vi "Get Label Prepend Append.vi"(8 "error in (no error)":errorcluster, 11 "CConfig Variant Accessor in":refnum<class "CConfig Variant Accessor.lvclass">) -> (0 "error out":errorcluster, 1 "Label Append":string, 2 "Label Prepend":string, 3 "CConfig Variant Accessor out":refnum<class "CConfig Variant Accessor.lvclass">)   [LabVIEW 2013, in "CConfig Variant Accessor.lvclass"]
doc: "Copyright 2018, Carya Automatisering, Wiebe Walstra."
uses:
  CConfig Variant Accessor.lvclass
  CConfig Variant Accessor.lvclass/CConfig Variant Accessor.ctl
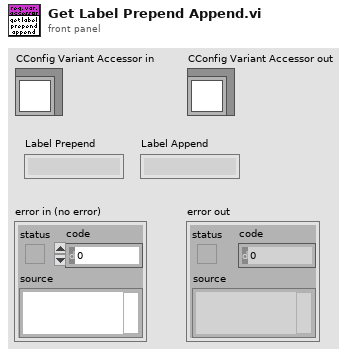
[diagram p1: front panel]
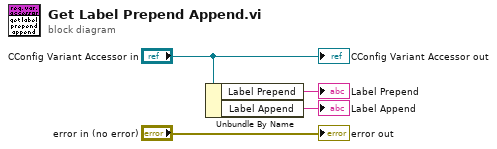
[diagram p0: block diagram]
diagram:
  n1 = Unbundle By Name("CConfig Variant Accessor in") -> ("Label Prepend"=→"Label Prepend":string, "Label Append"=→"Label Append":string)
  "error out" <- "error in (no error)"
  "CConfig Variant Accessor out" <- "CConfig Variant Accessor in"
